vi "9214_UI.vi"(8 "error in (no error)":errorcluster, 11 "Node Ptr":T5 format="%.0x") -> (0 "error out":errorcluster)   [LabVIEW 2017, in "Modules.lvlib" / "9214.lvclass"]
uses:
  9214.lvclass
  <vilib>/NI Veristand/Custom Device API/Custom Device Item Ref.ctl
  RSI Module/SubPanel Command.ctl
  9213/Channels Listbox.ctl
  9213/Thermocouple Type.ctl
  9213/Measurement Units.ctl
  9213/Conversion Time.ctl
  C:/Users/dbuck/Documents/GitHub/Scan-Engine-Custom-Device-Classes/Source/9213/9213.lvclass
  C:/Users/dbuck/Documents/GitHub/Scan-Engine-Custom-Device-Classes/Source/RSI Module/RSI Module.lvclass
  9214.lvclass/9214.ctl
  <vilib>/Utility/file.llb/Read From Spreadsheet File (DBL).vi
  <vilib>/Utility/file.llb/Write To Spreadsheet File (DBL).vi
  RSI Module/RSI Module.lvclass
  <vilib>/NI Veristand/Custom Device API/Custom Device API.lvlib
  9213/9213.lvclass
panel:
  in  "Export":bool
  in  "Import":bool
  in  "OTD compensation values":dbl[](array[numeric]) format="%#_21f"
  in  "OTDComp":bool
  in  "Conversion Time":T1=1 items=["High Speed", "High Resolution"]
  in  "Units":T2 caption="Measurement Units" items=["Raw Volts", "Degrees Kelvin", "Degrees Celsius", "Degrees Fahrenheit", "Degrees Rankine"]
  in  "Type":T3 caption="Thermocouple Type" items=["J", "K", "T", "E", "R", "S", "N", "B"]
  in  "Channels":T4=[0]
  in  "SubPanel Event":refnum<user-event>
  in  "Header":cluster{"Section Name":string}={"Section Name"="NI 9205 Settings"}
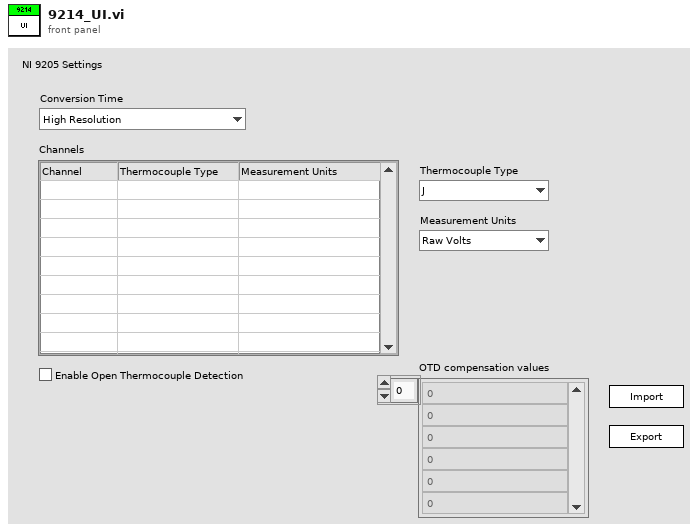
[diagram p1: front panel]
types:
  T1 = typedef "Modules.lvlib/9213.lvclass/Conversion Time.ctl" = u16
  T2 = typedef "Modules.lvlib/9213.lvclass/Measurement Units.ctl" = u8
  T3 = typedef "Modules.lvlib/9213.lvclass/Thermocouple Type.ctl" = u8
  T4 = typedef "Modules.lvlib/9213.lvclass/Channels Listbox.ctl" = i32[]
  T5 = typedef "Custom Device API.lvlib/Custom Device Item Ref.ctl" = u64
  T6 = enum8{"Enabled", "Disabled", "Disabled and Grayed Out"}
  T7 = typedef "Modules.lvlib/RSI Module.lvclass/Module Models.ctl" = enum16{"Empty", "NI 9201", "NI 9203", "NI 9205", "NI 9206", "NI 9207", "NI 9208", "NI 9211", "NI 9212", "NI 9213", "NI 9214", "NI 9215", "NI 9217", "NI 9219", "NI 9220", "NI 9221", "NI 9222", "NI 9223", "NI 9225", "NI 9227", "NI 9229", "NI 9233", "NI 9234", "NI 9235", "NI 9236", "NI 9237", "NI 9239", "NI 9242", "NI 9244", "NI 9263", "NI 9264", "NI 9265", "NI 9269", "NI 9375", "NI 9401", "NI 9402", "NI 9403", "NI 9411", "NI 9421", "NI 9422", "NI 9423", "NI 9425", "NI 9426", "NI 9435", "NI 9437", "NI 9472", "NI 9474", "NI 9475", "NI 9476", "NI 9477", "NI 9478", "NI 9481", "NI 9482", "NI 9485"}
  T8 = typedef "Modules.lvlib/RSI Module.lvclass/SubPanel Command.ctl" = enum16{"Stop"}
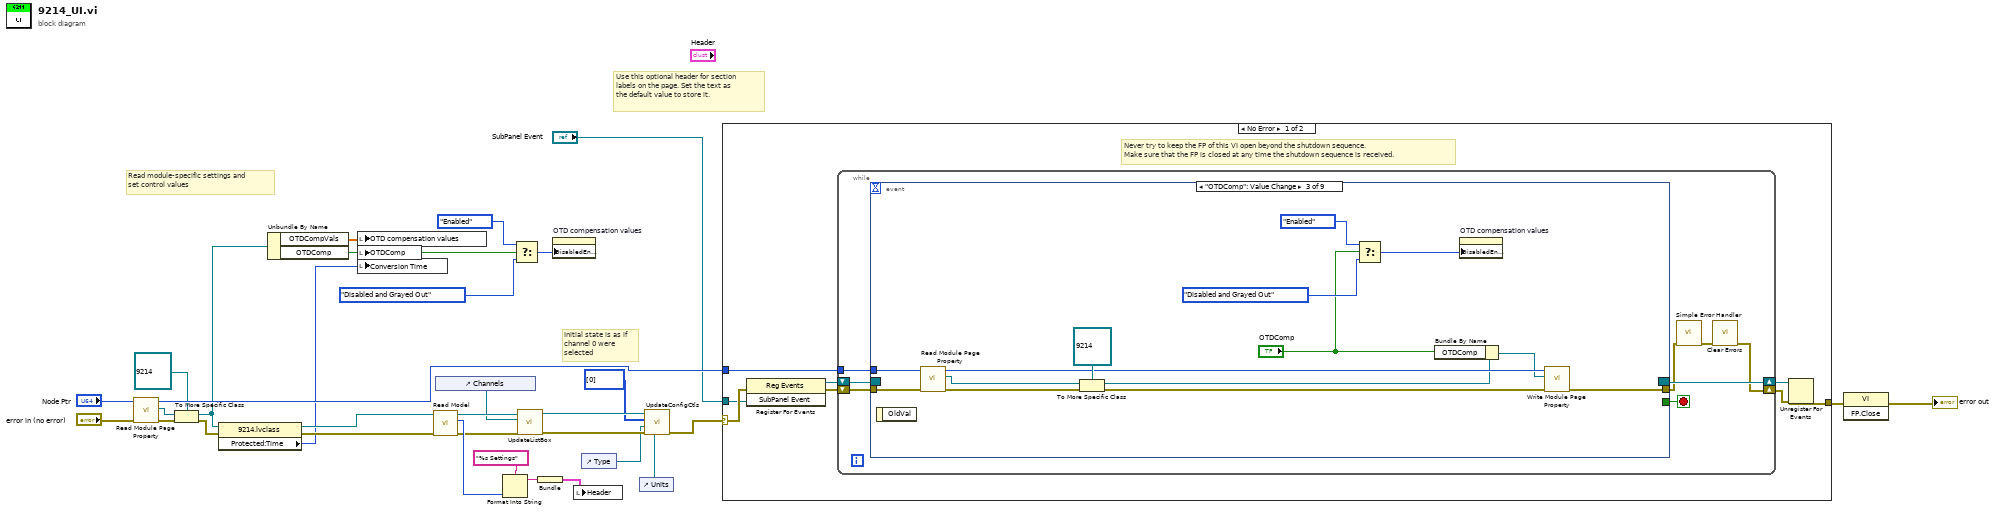
[diagram p0: block diagram]
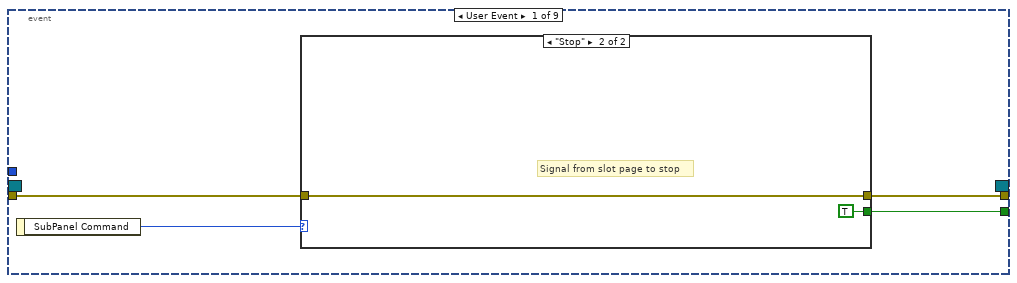
[diagram p2: hidden frame]
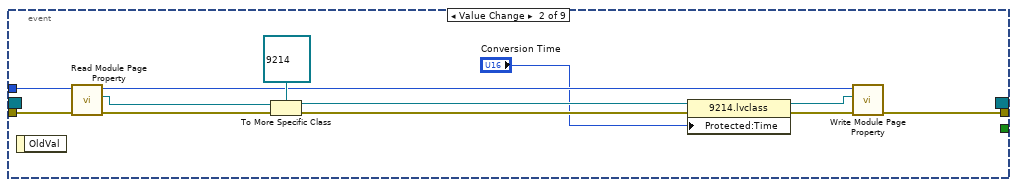
[diagram p4: hidden frame]
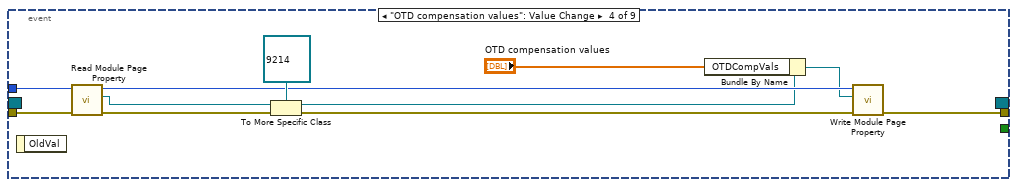
[diagram p5: hidden frame]
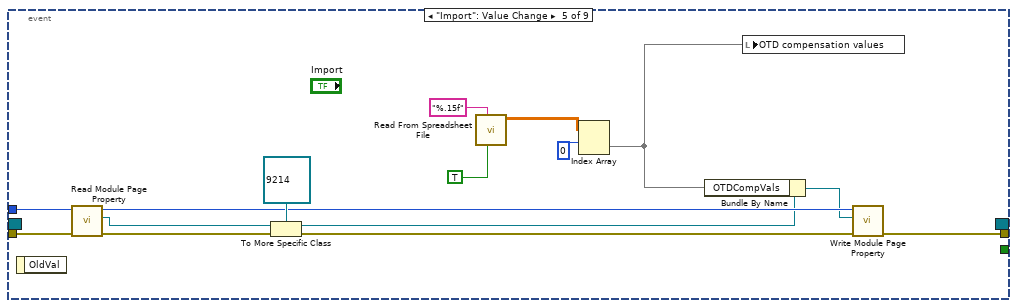
[diagram p6: hidden frame]
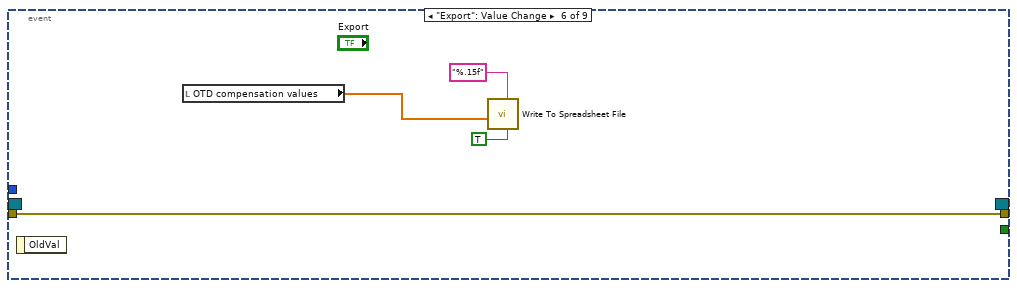
[diagram p7: hidden frame]
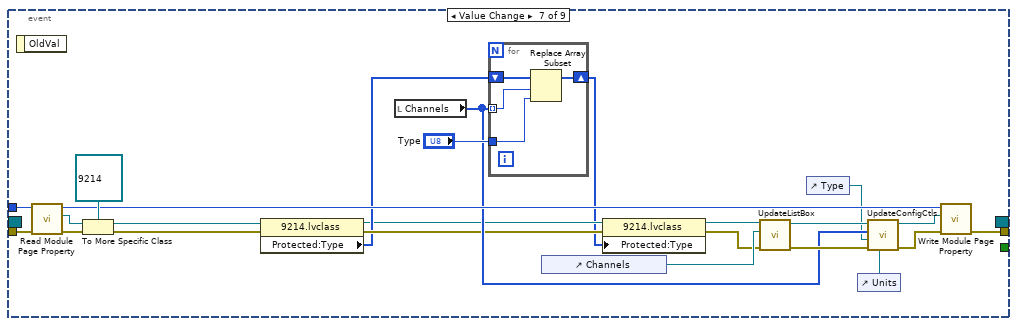
[diagram p8: hidden frame]
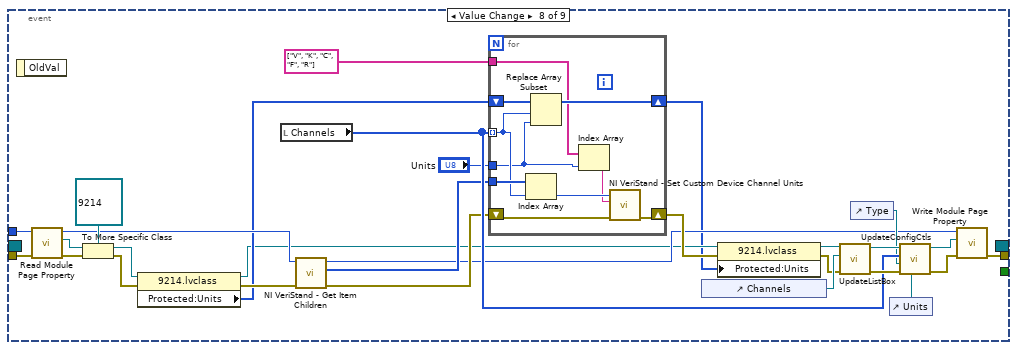
[diagram p9: hidden frame]
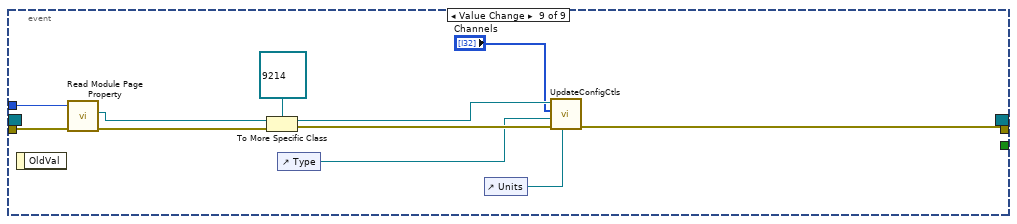
[diagram p10: hidden frame]
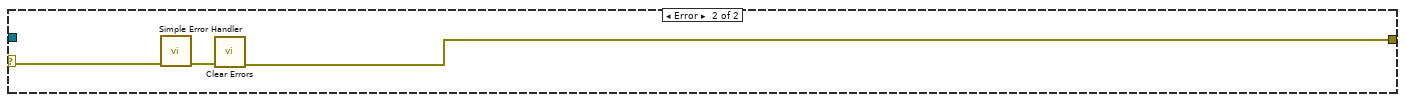
[diagram p11: hidden frame]
diagram:
  # "Initial state is as if channel 0 were selected"
  # "Read module-specific settings and\nset control values"
  # "Use this optional header for section labels on the page. Set the text as the default value to store it."
  n1 = call "Read Module Page Property.vi"("error in (no error)"="error in (no error)", "Node Ptr In"="Node Ptr") -> ("error out"=w26:errorcluster, "RSI Module"=w24:refnum<class "RSI Module.lvclass">, "Node Ptr Out"=w29:T5)  [unwired: 7 in]
  n2 = To More Specific Class(target class=refnum<class "9214.lvclass"> refnum ("9205 in"), reference=w24, error in=w26) -> (specific class reference=w3:refnum<class "9214.lvclass">, error out=w23:errorcluster)
  n3 = property class="9214.lvclass"(reference=w3, error in=w23) -> (reference out=w4:refnum<class "9214.lvclass">, error out=w5:errorcluster, "Protected:Time"=w2:T1)
  n4 = Unbundle By Name(w3) -> ("OTDCompVals"=w10:dbl[], "OTDComp"=w9:bool)
  n5 = local write "OTD compensation values"(w10) -> ()
  n6 = local write "OTDComp"(w9) -> ()
  n7 = local write "Conversion Time"(w2) -> ()
  n8 = call "Read Model.vi"("error in (no error)"=w5, "RSI Module in"=w4) -> ("error out"=w18:errorcluster, "Model"=w21:T7, "RSI Module out"=w17:refnum<class "9214.lvclass">)  [unwired: 7 in]
  n9 = control-ref of="Channels"() -> (w16:refnum<vi>)
  n10 = Format Into String(format string="%s Settings", w21) -> (resulting string=w19:string)  [unwired: 2 in, 1 out]
  n11 = Select(t=T6."Enabled" ("Disabled"), s=w9, f=T6."Disabled and Grayed Out" ("Disabled")) -> (s? t:f=w7:T6)
  n12 = call "UpdateListBox.vi"("error in (no error)"=w18, "ListBox Refnum"=w16, "9213 in"=w17) -> ("error out"=w15:errorcluster, "9213 out"=w14:refnum<class "9214.lvclass">)  [unwired: 7 in]
  n13 = Bundle(w19) -> (w22:cluster{string})  [unwired: 1 in]
  n14 = property on="OTD compensation values" class="Arr (strict)"("DisabledEnum"=w7) -> ()  [unwired: 2 in, 2 out]
  n15 = local write "Header"(w22) -> ()
  n16 = control-ref of="Type"() -> (w12:refnum<vi>)
  n17 = control-ref of="Units"() -> (w13:refnum<vi>)
  n18 = call "UpdateConfigCtls.vi"("Units"=w13, "error in (no error)"=w15, "Type"=w12, "Selected Channels"=T4 [0], "9213 in"=w14) -> ("error out"=w1:errorcluster)  [unwired: 5 in, 1 out]
  n19 = case shown="No Error" w1 {
    selector: w1 -> [w34 w192]
    tunnel: [w38 w190] -> w32
    tunnel: w29 -> [w35 _]
    tunnel: "SubPanel Event" -> [w33 _]
    frame No Error {
      # "Never try to keep the FP of this VI open beyond the shutdown sequence.\nMake sure that the FP is closed at any time the shutdown sequence is received."
      n20 = register-events(error in=w34, w33) -> (reference out=w36:refnum<event-registration>, error out=w37:errorcluster)  [unwired: 1 in]
      n21 = while {
        tunnel: w35 -> [w44]
        shift-right: [w41] -> w39
        shift-left: w37 -> [w47]
        shift-right: [w48] -> w40
        shift-left: w36 -> [w46]
        stop <- w45 stop-if-true
        n22 = event shown="[2] \"OTDComp\": Value Change" {
          selector: w46 -> [_ _ _ _ _ _ _ _ _]
          dyn-events: [_ _ _ _ _ _ _ _ _] -> w48
          timeout: _ -> [_ _ _ _ _ _ _ _ _]
          tunnel: w47 -> [w51 w61 w75 w86 w101 w111 w130 w164 w186]
          tunnel: [w50 _ _ _ _ _ _ _ _] -> w45
          tunnel: [w49 w60 w74 w85 w100 w111 w129 w163 w182] -> w43
          tunnel: w44 -> [_ w62 w76 w87 w102 _ w131 w165 w185]
          event User Event {
            n23 = event-data() -> ("SubPanel Command"=w52:T8)  [unwired: 1 out]
            n24 = case shown="\"Stop\"" w52 {
              tunnel: w51 -> [w53 w54]
              tunnel: [w53 w54] -> w49
              tunnel: [_ TRUE] -> w50
              frame Default {
              }
              frame "Stop" {
                # "Signal from slot page to stop"
              }
            }
          }
          event Value Change {
            n25 = event-data() -> ()  [unwired: 2 out]
            n26 = call "Read Module Page Property.vi"("error in (no error)"=w61, "Node Ptr In"=w62) -> ("error out"=w65:errorcluster, "RSI Module"=w66:refnum<class "RSI Module.lvclass">, "Node Ptr Out"=w63:T5)  [unwired: 7 in]
            n27 = To More Specific Class(target class=refnum<class "9214.lvclass"> refnum ("9205 in"), reference=w66, error in=w65) -> (specific class reference=w58:refnum<class "9214.lvclass">, error out=w64:errorcluster)
            n28 = property class="9214.lvclass"(reference=w58, error in=w64, "Protected:Time"="Conversion Time") -> (reference out=w56:refnum<class "9214.lvclass">, error out=w59:errorcluster)
            n29 = call "Write Module Page Property.vi"("error in (no error)"=w59, "RSI Module"=w56, "Node Ptr In"=w63) -> ("error out"=w60:errorcluster)  [unwired: 6 in, 2 out]
          }
          event "OTDComp": Value Change {
            n30 = event-data() -> ()  [unwired: 2 out]
            n31 = call "Read Module Page Property.vi"("error in (no error)"=w75, "Node Ptr In"=w76) -> ("error out"=w79:errorcluster, "RSI Module"=w80:refnum<class "RSI Module.lvclass">, "Node Ptr Out"=w77:T5)  [unwired: 7 in]
            n32 = To More Specific Class(target class=refnum<class "9214.lvclass"> refnum ("9205 in"), reference=w80, error in=w79) -> (specific class reference=w73:refnum<class "9214.lvclass">, error out=w78:errorcluster)
            n33 = Select(t=T6."Enabled" ("Disabled"), s="OTDComp", f=T6."Disabled and Grayed Out" ("Disabled")) -> (s? t:f=w70:T6)
            n34 = Bundle By Name(cluster=w73, "OTDComp"="OTDComp") -> (w72:refnum<class "9214.lvclass">)
            n35 = property on="OTD compensation values" class="Arr (strict)"("DisabledEnum"=w70) -> ()  [unwired: 2 in, 2 out]
            n36 = call "Write Module Page Property.vi"("error in (no error)"=w78, "RSI Module"=w72, "Node Ptr In"=w77) -> ("error out"=w74:errorcluster)  [unwired: 6 in, 2 out]
          }
          event "OTD compensation values": Value Change {
            n37 = event-data() -> ()  [unwired: 2 out]
            n38 = call "Read Module Page Property.vi"("error in (no error)"=w86, "Node Ptr In"=w87) -> ("error out"=w90:errorcluster, "RSI Module"=w91:refnum<class "RSI Module.lvclass">, "Node Ptr Out"=w88:T5)  [unwired: 7 in]
            n39 = To More Specific Class(target class=refnum<class "9214.lvclass"> refnum ("9205 in"), reference=w91, error in=w90) -> (specific class reference=w84:refnum<class "9214.lvclass">, error out=w89:errorcluster)
            n40 = Bundle By Name(cluster=w84, "OTDCompVals"="OTD compensation values") -> (w83:refnum<class "9214.lvclass">)
            n41 = call "Write Module Page Property.vi"("error in (no error)"=w89, "RSI Module"=w83, "Node Ptr In"=w88) -> ("error out"=w85:errorcluster)  [unwired: 6 in, 2 out]
          }
          event "Import": Value Change {
            n42 = event-data() -> ()  [unwired: 2 out]
            n43 = call "Read Module Page Property.vi"("error in (no error)"=w101, "Node Ptr In"=w102) -> ("error out"=w105:errorcluster, "RSI Module"=w106:refnum<class "RSI Module.lvclass">, "Node Ptr Out"=w103:T5)  [unwired: 7 in]
            n44 = To More Specific Class(target class=refnum<class "9214.lvclass"> refnum ("9205 in"), reference=w106, error in=w105) -> (specific class reference=w99:refnum<class "9214.lvclass">, error out=w104:errorcluster)
            n45 = call-poly <vilib>:"Read From Spreadsheet File.vi"("transpose (no:F)"=TRUE, "format (%.3f)"="%.15f" ("format string")) -> ("all rows"=w96:dbl[][])  [unwired: 5 in, 4 out]
            n46 = Index Array(array=w96, index (row)=0 ("disabled index (col)")) -> (element=w95:dbl[])  [unwired: 1 in]
            n47 = Bundle By Name(cluster=w99, "OTDCompVals"=w95) -> (w98:refnum<class "9214.lvclass">)
            n48 = local write "OTD compensation values"(w95) -> ()
            n49 = call "Write Module Page Property.vi"("error in (no error)"=w104, "RSI Module"=w98, "Node Ptr In"=w103) -> ("error out"=w100:errorcluster)  [unwired: 6 in, 2 out]
          }
          event "Export": Value Change {
            n50 = event-data() -> ()  [unwired: 2 out]
            n51 = local read "OTD compensation values"() -> (w109:dbl[])
            n52 = call-poly <vilib>:"Write To Spreadsheet File.vi"("transpose? (no:F)"=TRUE, "format (%.3f)"="%.15f", "1D data"=w109) -> ()  [unwired: 5 in, 1 out]
          }
          event Value Change {
            n53 = event-data() -> ()  [unwired: 2 out]
            n54 = call "Read Module Page Property.vi"("error in (no error)"=w130, "Node Ptr In"=w131) -> ("error out"=w133:errorcluster, "RSI Module"=w134:refnum<class "RSI Module.lvclass">, "Node Ptr Out"=w132:T5)  [unwired: 7 in]
            n55 = To More Specific Class(target class=refnum<class "9214.lvclass"> refnum ("9205 in"), reference=w134, error in=w133) -> (specific class reference=w117:refnum<class "9214.lvclass">, error out=w127:errorcluster)
            n56 = property class="9214.lvclass"(reference=w117, error in=w127) -> (reference out=w114:refnum<class "9214.lvclass">, error out=w118:errorcluster, "Protected:Type"=w116:T3[])
            n57 = local read "Channels"() -> (w123:T4)
            n58 = for {
              tunnel: w123 -> [w137] mode=indexing
              shift-right: [w138] -> w112
              shift-left: w116 -> [w139]
              tunnel: "Type" -> [w136]
              n59 = Replace Array Subset(array=w139, new element=w136, index=w137) -> (w138:T3[])
            }
            n60 = control-ref of="Channels"() -> (w122:refnum<vi>)
            n61 = property class="9214.lvclass"(reference=w114, error in=w118, "Protected:Type"=w112) -> (reference out=w113:refnum<class "9214.lvclass">, error out=w115:errorcluster)
            n62 = call "UpdateListBox.vi"("error in (no error)"=w115, "ListBox Refnum"=w122, "9213 in"=w113) -> ("error out"=w126:errorcluster, "9213 out"=w124:refnum<class "9214.lvclass">)  [unwired: 7 in]
            n63 = control-ref of="Type"() -> (w120:refnum<vi>)
            n64 = control-ref of="Units"() -> (w121:refnum<vi>)
            n65 = call "UpdateConfigCtls.vi"("Units"=w121, "error in (no error)"=w126, "Type"=w120, "Selected Channels"=w123, "9213 in"=w124) -> ("error out"=w125:errorcluster, "9213 out"=w119:refnum<class "9214.lvclass">)  [unwired: 5 in]
            n66 = call "Write Module Page Property.vi"("error in (no error)"=w125, "RSI Module"=w119, "Node Ptr In"=w132) -> ("error out"=w129:errorcluster)  [unwired: 6 in, 2 out]
          }
          event Value Change {
            n67 = event-data() -> ()  [unwired: 2 out]
            n68 = call "Read Module Page Property.vi"("error in (no error)"=w164, "Node Ptr In"=w165) -> ("error out"=w166:errorcluster, "RSI Module"=w167:refnum<class "RSI Module.lvclass">, "Node Ptr Out"=w152:T5)  [unwired: 7 in]
            n69 = To More Specific Class(target class=refnum<class "9214.lvclass"> refnum ("9205 in"), reference=w167, error in=w166) -> (specific class reference=w145:refnum<class "9214.lvclass">, error out=w153:errorcluster)
            n70 = property class="9214.lvclass"(reference=w145, error in=w153) -> (reference out=w142:refnum<class "9214.lvclass">, error out=w146:errorcluster, "Protected:Units"=w144:T2[])
            n71 = local read "Channels"() -> (w159:T4)
            n72 = call <vilib>:"NI VeriStand - Get Item Children.vi"("error in (no error)"=w146, "Item Ref in"=w152) -> ("error out"=w150:errorcluster, "Child Refs"=w151:T5[], "Item Ref out"=w147:T5)  [unwired: 6 in, 1 out]
            n73 = for {
              tunnel: w159 -> [w175] mode=indexing
              shift-right: [w177] -> w140
              shift-left: w144 -> [w178]
              tunnel: "Units" -> [w170]
              shift-right: [w172] -> w149
              shift-left: w150 -> [w173]
              tunnel: w151 -> [w176]
              tunnel: string[] ["V", "K", "C", "F", "R"] -> [w171]
              n74 = Index Array(array=w176, index=w175) -> (element=w174:T5)
              n75 = Replace Array Subset(array=w178, new element=w170, index=w175) -> (w177:T2[])
              n76 = Index Array(array=w171, index=w170) -> (element=w169:string)
              n77 = call <vilib>:"NI VeriStand - Set Custom Device Channel Units.vi"("error in (no error)"=w173, "Units"=w169, "Channel Ref in"=w174) -> ("error out"=w172:errorcluster)  [unwired: 7 in, 1 out]
            }
            n78 = control-ref of="Channels"() -> (w158:refnum<vi>)
            n79 = property class="9214.lvclass"(reference=w142, error in=w149, "Protected:Units"=w140) -> (reference out=w141:refnum<class "9214.lvclass">, error out=w143:errorcluster)
            n80 = call "UpdateListBox.vi"("error in (no error)"=w143, "ListBox Refnum"=w158, "9213 in"=w141) -> ("error out"=w162:errorcluster, "9213 out"=w160:refnum<class "9214.lvclass">)  [unwired: 7 in]
            n81 = control-ref of="Type"() -> (w155:refnum<vi>)
            n82 = control-ref of="Units"() -> (w157:refnum<vi>)
            n83 = call "UpdateConfigCtls.vi"("Units"=w157, "error in (no error)"=w162, "Type"=w155, "Selected Channels"=w159, "9213 in"=w160) -> ("error out"=w161:errorcluster, "9213 out"=w154:refnum<class "9214.lvclass">)  [unwired: 5 in]
            n84 = call "Write Module Page Property.vi"("error in (no error)"=w161, "RSI Module"=w154, "Node Ptr In"=w147) -> ("error out"=w163:errorcluster)  [unwired: 6 in, 2 out]
          }
          event Value Change {
            n85 = event-data() -> ()  [unwired: 2 out]
            n86 = call "Read Module Page Property.vi"("error in (no error)"=w186, "Node Ptr In"=w185) -> ("error out"=w187:errorcluster, "RSI Module"=w188:refnum<class "RSI Module.lvclass">)  [unwired: 7 in, 1 out]
            n87 = To More Specific Class(target class=refnum<class "9214.lvclass"> refnum ("9205 in"), reference=w188, error in=w187) -> (specific class reference=w183:refnum<class "9214.lvclass">, error out=w184:errorcluster)
            n88 = control-ref of="Type"() -> (w180:refnum<vi>)
            n89 = control-ref of="Units"() -> (w181:refnum<vi>)
            n90 = call "UpdateConfigCtls.vi"("Units"=w181, "error in (no error)"=w184, "Type"=w180, "Selected Channels"="Channels", "9213 in"=w183) -> ("error out"=w182:errorcluster)  [unwired: 5 in, 1 out]
          }
        }
        n91 = call <vilib>:"Simple Error Handler.vi"("error in (no error)"=w43) -> ("error out"=w42:errorcluster)  [unwired: 1 in, 7 out]
        n92 = call <vilib>:"Clear Errors.vi"("error in (no error)"=w42) -> ("error out"=w41:errorcluster)  [unwired: 1 in, 5 out]
      }
      n93 = Unregister For Events(event registration refnum=w40, error in=w39) -> (error out=w38:errorcluster)
    }
    frame Error {
      n94 = call <vilib>:"Simple Error Handler.vi"("error in (no error)"=w192) -> ("error out"=w191:errorcluster)  [unwired: 1 in, 7 out]
      n95 = call <vilib>:"Clear Errors.vi"("error in (no error)"=w191) -> ("error out"=w190:errorcluster)  [unwired: 1 in, 5 out]
    }
  }
  n96 = invoke class="VI" method="FP.Close"(error in=w32) -> (error out=→"error out":errorcluster)  [unwired: 2 in, 2 out]
